vi "Leer.vi"() -> ()   [LabVIEW 2021]
uses:
  <vilib>/Utility/error.llb/DialogType.ctl
  <vilib>/Utility/file.llb/Read Delimited Spreadsheet (string).vi
  Global 1.vi
  <vilib>/Utility/file.llb/Write Delimited Spreadsheet (string).vi
panel:
  out "Sensor de presión":dynamicdata(graph)
  out "Trabajando":bool
  in  "Grabar":bool
  out "Archivo a generar":string
  in  "stop 2":bool
  out "Experimento Nº":i16=1
  out "Tipo":string
  out "Regulador de presión":dynamicdata(graph)
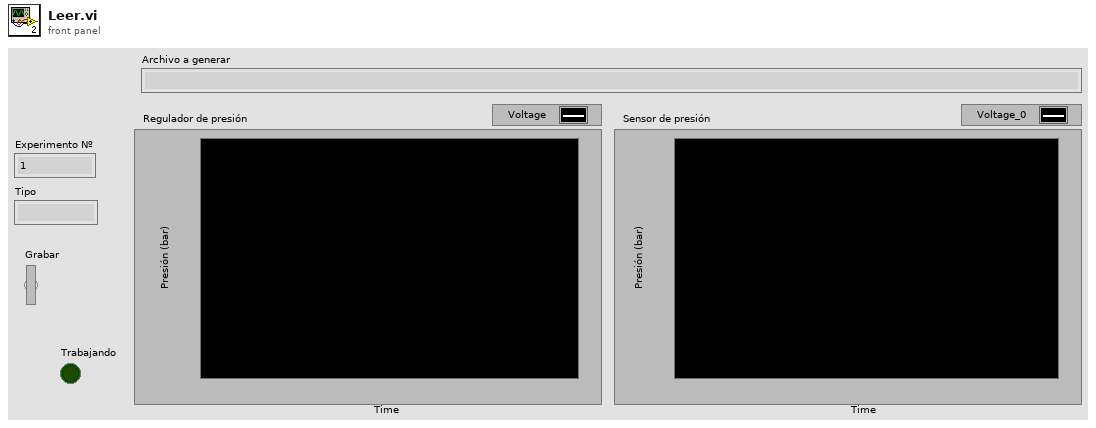
[diagram p1: front panel]
types:
  T1 = typedef "DialogType.ctl" = u16
  T2 = typedef "NI_Matrix.lvlib/RealMatrix.ctl" = dbl[][]
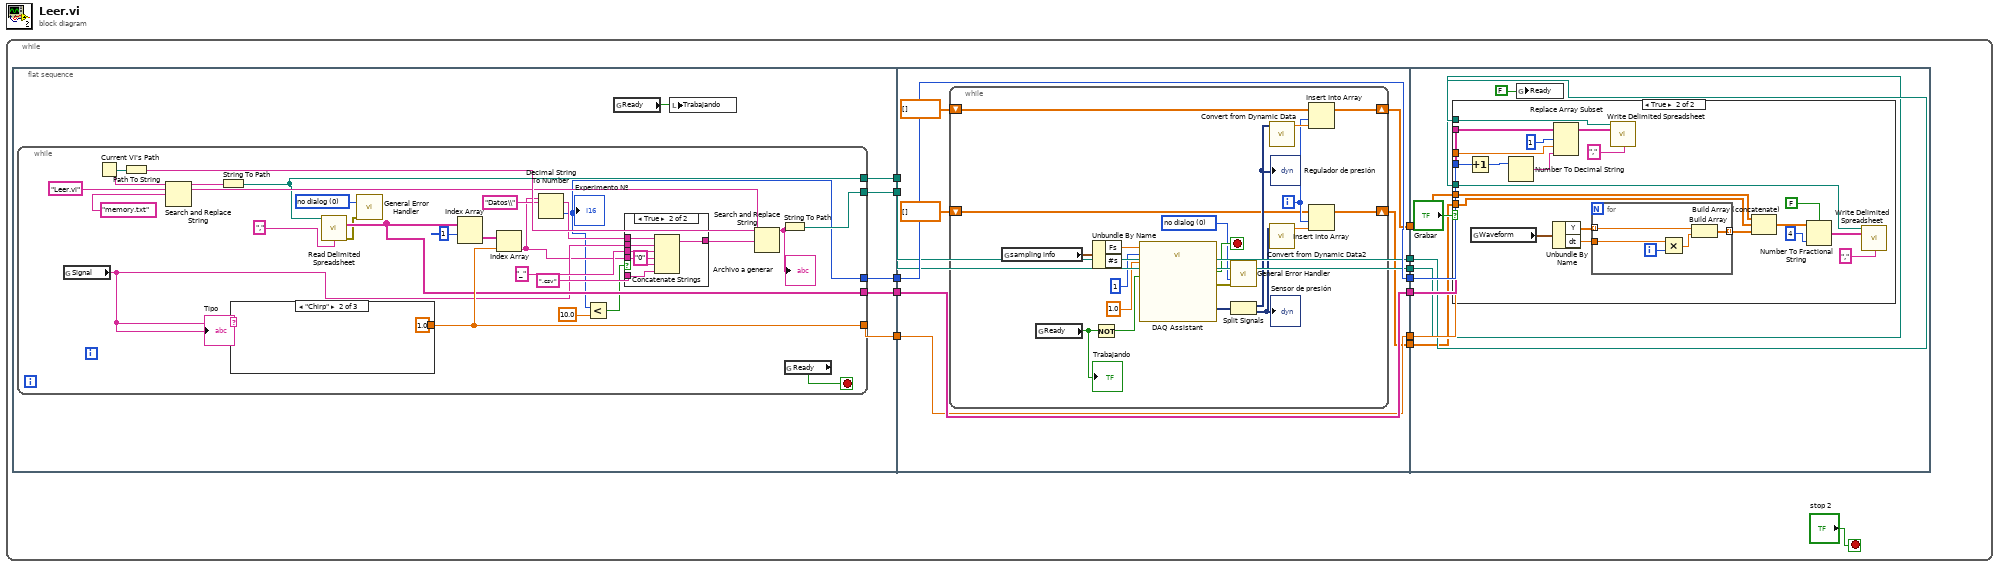
[diagram p0: block diagram]
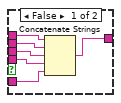
[diagram p2: hidden frame]
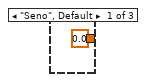
[diagram p3: hidden frame]
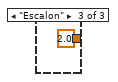
[diagram p4: hidden frame]
diagram:
  n1 = while {
    stop <- "stop 2" stop-if-true
    n2 = flat-sequence {
      tunnel: [w19] -> w12
      tunnel: [w18] -> w11
      tunnel: [w17] -> w8
      tunnel: [w16] -> w5
      tunnel: [w15] -> w4
      tunnel: [w69] -> w10
      tunnel: [w68] -> w9
      tunnel: [w67] -> w7
      tunnel: [w66] -> w6
      tunnel: w5 -> [w66]
      tunnel: w8 -> [w68]
      tunnel: w11 -> [w69]
      tunnel: w12 -> [w67]
      tunnel: w4 -> [w65]
      tunnel: [w65] -> w3
      tunnel: [w64] -> w2
      tunnel: [w61] -> w1
      tunnel: w10 -> [w97]
      tunnel: w9 -> [w96]
      tunnel: w7 -> [w95]
      tunnel: w6 -> [w94]
      tunnel: w3 -> [w92]
      tunnel: w2 -> [w90]
      tunnel: w1 -> [w89]
      frame #0 {
        n3 = while {
          tunnel: [w35] -> w19
          tunnel: [w20] -> w18
          tunnel: [w34] -> w17
          tunnel: [w33] -> w16
          tunnel: [w28] -> w15
          stop <- w38 stop-if-true
          w23 = T1 0 items=["no dialog", "OK message", "continue or stop message", "OK message + warnings", "continue/stop + warnings"] ("type of dialog (OK msg:1)")
          w42 = "Leer.vi" ("substring (\"\")")
          n4 = global read "Global 1.vi" "Signal"() -> (w26:string)
          "Tipo" <- w26
          n5 = Current VI's Path() -> (path=w44:path)
          n6 = Path To String(path=w44) -> (string=w43:string)
          n7 = Search and Replace String(input string=w43, search string=w42, replace string="memory.txt" ("replace string (\"\")")) -> (result string=w40:string)  [unwired: 5 in, 3 out]
          n8 = String To Path(string=w40) -> (path=w33:path)
          n9 = case shown="\"Chirp\"" w26 {
            tunnel: [0.0 ("x") 1.0 ("x") 2.0 ("x")] -> w35
            frame "Seno", Default {
            }
            frame "Chirp" {
            }
            frame "Escalon" {
            }
          }
          n10 = call-poly <vilib>:"Read Delimited Spreadsheet.vi"("file path (dialog if empty)"=w33, "delimiter (\\t)"="," ("delimiter (\\t)")) -> ("all rows"=w34:string[][], "error out"=w24:errorcluster)  [unwired: 8 in, 4 out]
          n11 = call <vilib>:"General Error Handler.vi"("type of dialog (OK msg:1)"=w23, "error in (no error)"=w24) -> ()  [unwired: 9 in, 5 out]
          n12 = Index Array(array=w34, index (row)=1) -> (element=w36:string[])  [unwired: 1 in]
          n13 = Index Array(array=w36, index=w35) -> (element=w25:string)
          n14 = Decimal String To Number(string=w25) -> (number=w20:i32)  [unwired: 2 in, 1 out]
          "Experimento Nº" <- w20
          n15 = Less?(x=w20, y=10.0) -> (x < y?=w21:bool)
          n16 = case shown="True" w21 {
            tunnel: "_" ("string") -> [w47 w57]
            tunnel: "Datos\\" ("replace string (\"\")") -> [w49 w56]
            tunnel: [w50 w55] -> w30
            tunnel: ".csv" ("string") -> [w45 w53]
            tunnel: w26 -> [w48 w54]
            tunnel: w25 -> [w46 w52]
            frame False {
              n17 = Concatenate Strings(w49, w48, w47, w46, w45) -> (w50:string)
            }
            frame True {
              n18 = Concatenate Strings(w56, w54, w57, "0" ("string"), w52, w53) -> (w55:string)
            }
          }
          n19 = Search and Replace String(input string=w43, search string=w42, replace string=w30) -> (result string=w29:string)  [unwired: 5 in, 3 out]
          "Archivo a generar" <- w29
          n20 = String To Path(string=w29) -> (path=w28:path)
          n21 = global read "Global 1.vi" "Ready"() -> (w38:bool)
        }
        n22 = global read "Global 1.vi" "Ready"() -> (w14:bool)
        n23 = local write "Trabajando"(w14) -> ()
      }
      frame #1 {
        n24 = while {
          shift-right: [w83] -> w64
          shift-left: dbl[] [] -> [w82]
          shift-right: [w70] -> w61
          shift-left: dbl[] [] -> [w71]
          i -> [w72]
          stop <- w86 stop-if-true
          w84 = T1 0 items=["no dialog", "OK message", "continue or stop message", "OK message + warnings", "continue/stop + warnings"] ("type of dialog (OK msg:1)")
          n25 = global read "Global 1.vi" "sampling info"() -> (w88:cluster{"Fs":dbl, "#s":dbl})
          n26 = global read "Global 1.vi" "Ready"() -> (w87:bool)
          "Trabajando" <- w87
          n27 = Unbundle By Name(w88) -> ("Fs"=w80:dbl)  [unwired: 1 out]
          n28 = Not(x=w87) -> (.not. x?=w78:bool)
          n29 = call "DAQ Assistant"("rate"=w80, "number of samples"=1, "timeout (s)"=1.0, "stop (F)"=w78) -> ("data"=w76:dynamicdata, "stopped"=w86:bool, "error out"=w85:errorcluster)  [unwired: 12 in, 1 out]
          n30 = call <vilib>:"General Error Handler.vi"("type of dialog (OK msg:1)"=w84, "error in (no error)"=w85) -> ()  [unwired: 9 in, 5 out]
          n31 = Split Signals(w76) -> (w75:dynamicdata, w73:dynamicdata)  [unwired: 2 in]
          "Regulador de presión" <- w75
          "Sensor de presión" <- w73
          n32 = call "Convert from Dynamic Data"("Dynamic Data Type"=w75) -> ("Scalar"=w81:dbl)  [unwired: 3 in]
          n33 = call "Convert from Dynamic Data2"("Dynamic Data Type"=w73) -> ("Scalar"=w74:dbl)  [unwired: 3 in]
          n34 = Insert Into Array(array=w82, index=w72, new element=w81) -> (w83:dbl[])
          n35 = Insert Into Array(array=w71, index=w72, new element=w74) -> (w70:dbl[])
        }
      }
      frame #2 {
        n36 = case shown="True" "Grabar" {
          tunnel: w97 -> [_ w117]
          tunnel: w96 -> [_ w116]
          tunnel: w95 -> [_ w114]
          tunnel: w94 -> [_ w112]
          tunnel: w92 -> [_ w109]
          tunnel: w90 -> [_ w100]
          tunnel: w89 -> [_ w98]
          frame False {
          }
          frame True {
            n37 = Increment(x=w117) -> (x+1=w118:i32)
            n38 = global read "Global 1.vi" "Waveform"() -> (w108:waveform(dbl))
            n39 = Number To Decimal String(number=w118) -> (decimal integer string=w113:string)  [unwired: 1 in]
            n40 = Unbundle By Name(w108) -> ("Y"=w106:dbl[], "dt"=w107:dbl)
            n41 = Replace Array Subset(array=w116, new element=w113, index (row)=1, index (col)=w114) -> (w111:string[][])
            n42 = for {
              tunnel: w106 -> [w120] mode=indexing
              tunnel: w107 -> [w122]
              tunnel: [w119] -> w99 mode=indexing
              i -> [w123]
              n43 = Multiply(x=w122, y=w123) -> (x*y=w121:dbl)
              n44 = Build Array(w120, w121) -> (w119:dbl[])
            }
            n45 = call-poly <vilib>:"Write Delimited Spreadsheet.vi"("file path (dialog if empty)"=w112, "2D data"=w111, "delimiter (\\t)"="," ("delimiter (\\t)")) -> ()  [unwired: 11 in, 2 out]
            n46 = Build Array (concatenate)(w100, w98, w99) -> (w101:T2)
            n47 = Number To Fractional String(use system decimal point (T)=FALSE, number=w101, precision (6)=i16 4) -> (F-format string=w102:string[][])  [unwired: 1 in]
            n48 = call-poly <vilib>:"Write Delimited Spreadsheet.vi"("file path (dialog if empty)"=w109, "2D data"=w102, "delimiter (\\t)"="," ("delimiter (\\t)")) -> ()  [unwired: 11 in, 2 out]
          }
        }
        n49 = global write "Global 1.vi" "Ready"(FALSE ("Ready")) -> ()
      }
    }
  }
